vi "Calculate Constants.vi"(1 "Axes Magnitudes":cluster{"X":dbl, "Y":dbl, "Z":dbl}, 2 "Length/2":dbl=0.4359402 format="%#_13g", 3 "Width/2":dbl=0.5588 format="%#_13g") -> (0 "constants cluster":cluster{"a":dbl, "b":dbl, "c":dbl, "d":dbl})   [LabVIEW 2016, in "Huskie Swerve.lvlib"]
uses:
  Huskie Swerve.lvlib
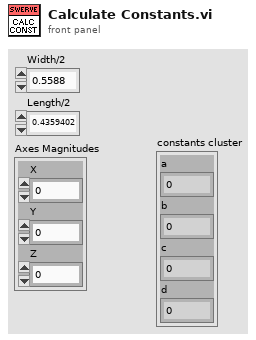
[diagram p1: front panel]
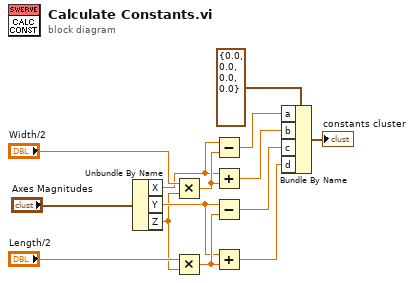
[diagram p0: block diagram]
diagram:
  n1 = Unbundle By Name("Axes Magnitudes") -> ("X"=w3:dbl, "Y"=w2:dbl, "Z"=w1:dbl)
  n2 = Multiply(x="Width/2", y=w1) -> (x*y=w5:dbl)
  n3 = Multiply(x="Length/2", y=w1) -> (x*y=w7:dbl)
  n4 = Subtract(x=w3, y=w5) -> (x-y=w12:dbl)
  n5 = Add(x=w3, y=w5) -> (x+y=w10:dbl)
  n6 = Subtract(x=w2, y=w7) -> (x-y=w8:dbl)
  n7 = Add(x=w2, y=w7) -> (x+y=w6:dbl)
  n8 = Bundle By Name(cluster=cluster{"a":dbl, "b":dbl, "c":dbl, "d":dbl} {"a"=0.0, "b"=0.0, "c"=0.0, "d"=0.0}, "a"=w12, "b"=w10, "c"=w8, "d"=w6) -> (→"constants cluster":cluster{"a":dbl, "b":dbl, "c":dbl, "d":dbl})
